vi "Select Lamp.vi"(8 "error in (no error)":errorcluster {"code" format="%.0x"}, 9 "Lamp Type (0: Transmitted)":enum16{"Transmitted", "Reflected"}(ring), 10 "Device Number (1)":i32=1, 11 "VISA Resource Name":refnum<visa-resource-name>) -> (0 "error out":errorcluster {"code" format="%.0x"}, 3 "VISA Resource Name Out":refnum<visa-resource-name>)   [LabVIEW 2020, in "Olympus IX BX Series.lvlib"]
doc: "Select the lamps for reflected light / transmitted light (for DIA/EPI)."
uses:
  Olympus IX BX Series.lvlib
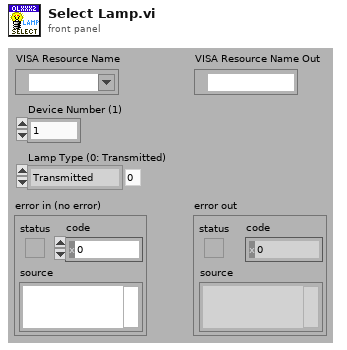
[diagram p1: front panel]
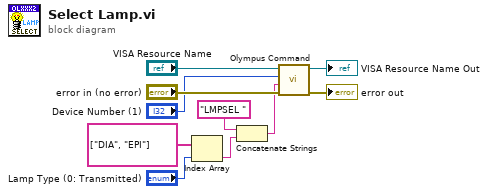
[diagram p0: block diagram]
diagram:
  n1 = Index Array(array=string[] ["DIA", "EPI"], index="Lamp Type (0: Transmitted)") -> (element=w3:string)
  n2 = Concatenate Strings("LMPSEL ", w3) -> (w2:string)
  n3 = call "Olympus Command.vi"("error in (no error)"="error in (no error)", "Command string"=w2, "Device Number (1)"="Device Number (1)", "VISA Resource Name"="VISA Resource Name") -> ("error out"=→"error out":errorcluster, "VISA Resource Name Out"=→"VISA Resource Name Out":refnum<visa-resource-name>)  [unwired: 5 in, 1 out]
